vi "Event data  Queues Manager.vi"(0 "event":string, 1 "Mode":T1, 5 "Message":string, 7 "Time Stamp":timestamp, 9 "data":string, 11 "error in":errorcluster, 12 "Front?":bool) -> (6 "process":cluster{"event":string, "par":string}, 8 "data":cluster{"time":timestamp, "data":string}, 10 "timed out?":bool, 15 "error out":errorcluster)   [LabVIEW 2015, in "event data queues.lvlib"]
doc: "Use this template to build a VI to use as a subVI."
uses:
  event data queues.lvlib
  Enum data queue_Ctrls.ctl
panel:
  in  "queues":T2
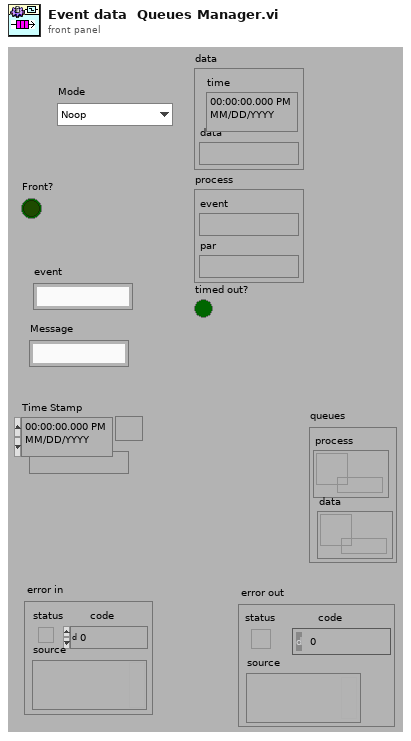
[diagram p1: front panel]
types:
  T1 = typedef "event data queues.lvlib/Enum data queue_Ctrls.ctl" = enum16{"Noop", "Send Pro1", "Send data", "Get Pro1", "Get data", "Flush Pro1", "Flush data", "Destroy Pro1", "Destroy data"}
  T2 = cluster{"process":refnum<queue>, "data":refnum<queue>}
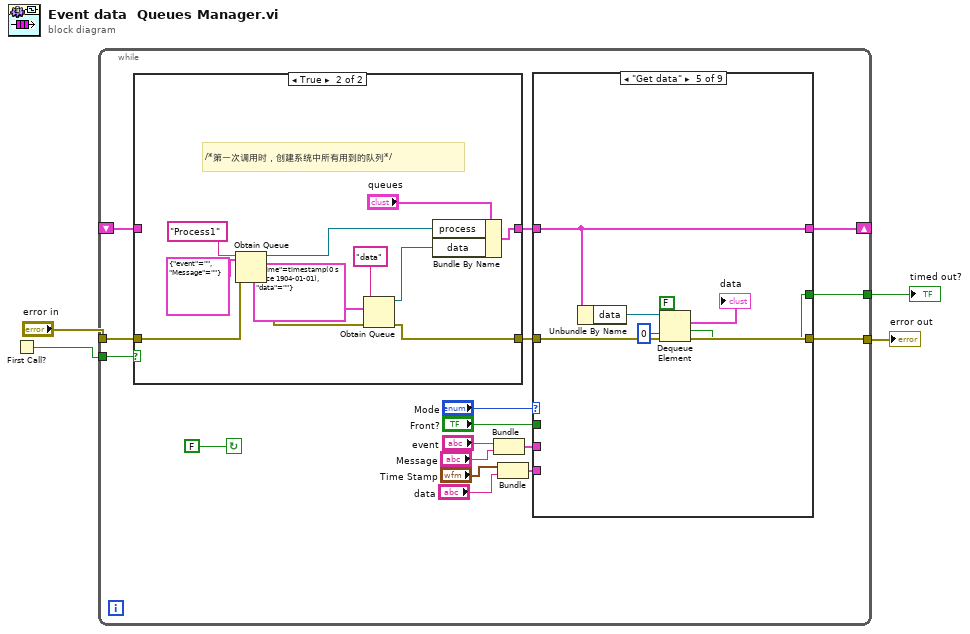
[diagram p0: block diagram]
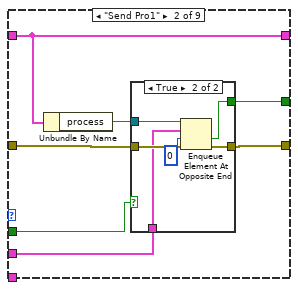
[diagram p3: hidden frame]
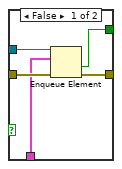
[diagram p4: hidden frame]
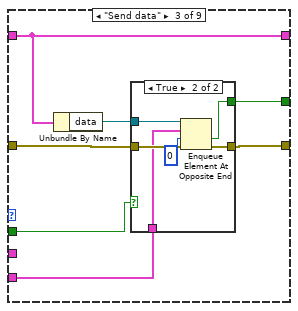
[diagram p5: hidden frame]
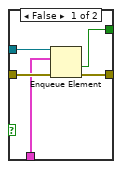
[diagram p6: hidden frame]
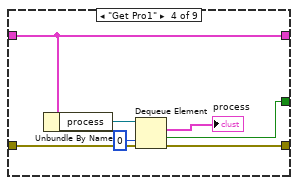
[diagram p7: hidden frame]
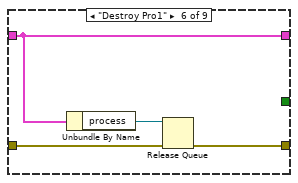
[diagram p8: hidden frame]
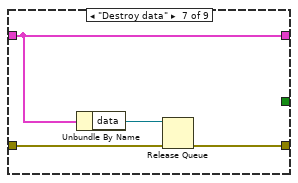
[diagram p9: hidden frame]
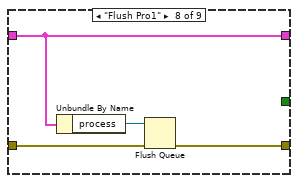
[diagram p10: hidden frame]
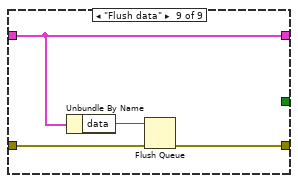
[diagram p11: hidden frame]
diagram:
  n1 = First Call?() -> (First Call?: T/F=w4:bool)
  n2 = while {
    tunnel: w4 -> [w20]
    tunnel: [w16] -> w2
    shift-right: [w15] -> _
    shift-left: _ -> [w14]
    tunnel: "error in" -> [w13]
    tunnel: [w5] -> w1
    stop <- FALSE continue-if-true
    n3 = case shown="True" w20 {
      tunnel: [w91 w100] -> w18
      tunnel: [w90 w97] -> w17
      tunnel: w14 -> [w91 _]
      tunnel: w13 -> [w90 w98]
      frame False {
      }
      frame True {
        # "/*第一次调用时，创建系统中所有用到的队列*/"
        n4 = Obtain Queue(name (unnamed)="Process1", element data type=cluster{"event":string, "Message":string} {"event"="", "Message"=""} ("Cluster"), error in (no error)=w98) -> (queue out=w93:refnum<queue>, error out=w94:errorcluster)  [unwired: 2 in, 1 out]
        n5 = Obtain Queue(name (unnamed)="data", element data type=cluster{"time":timestamp, "data":string} {"time"=timestamp(0 s since 1904-01-01), "data"=""} ("Cluster"), error in (no error)=w94) -> (queue out=w92:refnum<queue>, error out=w97:errorcluster)  [unwired: 2 in, 1 out]
        n6 = Bundle By Name(cluster="queues", "process"=w93, "data"=w92) -> (w100:T2)
      }
    }
    n7 = Bundle("event"="event", "Message"="Message") -> (w11:cluster{"event":string, "Message":string})  [unwired: 1 out]
    n8 = Bundle("Time Stamp"="Time Stamp", "data"="data") -> (w9:cluster{"Time Stamp":timestamp, "data":string})  [unwired: 1 out]
    n9 = case shown="\"Get data\"" "Mode" {
      tunnel: w18 -> [w23 w28 w46 w63 w70 w74 w78 w84 w88]
      tunnel: w17 -> [w22 w30 w48 w65 w72 w77 w81 w83 w87]
      tunnel: [w22 w29 w47 w64 w71 w76 w80 w82 w86] -> w16
      tunnel: [w23 w28 w46 w63 w70 w74 w78 w84 w88] -> w15
      tunnel: "Front?" -> [_ w27 w45 _ _ _ _ _ _]
      tunnel: w11 -> [_ w25 _ _ _ _ _ _ _]
      tunnel: w9 -> [_ _ w43 _ _ _ _ _ _]
      tunnel: [_ w24 w42 w60 w67 _ _ _ _] -> w5
      frame "Noop", Default {
      }
      frame "Send Pro1" {
        n10 = Unbundle By Name(w28) -> ("process"=w26:refnum<queue>)
        n11 = case shown="True" w27 {
          tunnel: w30 -> [w35 w41]
          tunnel: [w34 w40] -> w29
          tunnel: w26 -> [w33 w38]
          tunnel: w25 -> [w32 w37]
          tunnel: [w31 w36] -> w24
          frame False {
            n12 = Enqueue Element(queue=w33, element=w32, error in (no error)=w35) -> (timed out?=w31:bool, error out=w34:errorcluster)  [unwired: 2 out]
          }
          frame True {
            n13 = Enqueue Element At Opposite End(queue=w38, element=w37, timeout in ms (-1)=0, error in (no error)=w41) -> (timed out?=w36:bool, error out=w40:errorcluster)  [unwired: 1 out]
          }
        }
      }
      frame "Send data" {
        n14 = Unbundle By Name(w46) -> ("data"=w44:refnum<queue>)
        n15 = case shown="True" w45 {
          tunnel: w48 -> [w53 w59]
          tunnel: [w52 w58] -> w47
          tunnel: w44 -> [w51 w56]
          tunnel: w43 -> [w50 w55]
          tunnel: [w49 w54] -> w42
          frame False {
            n16 = Enqueue Element(queue=w51, element=w50, error in (no error)=w53) -> (timed out?=w49:bool, error out=w52:errorcluster)  [unwired: 1 in, 1 out]
          }
          frame True {
            n17 = Enqueue Element At Opposite End(queue=w56, element=w55, timeout in ms (-1)=0, error in (no error)=w59) -> (timed out?=w54:bool, error out=w58:errorcluster)  [unwired: 1 out]
          }
        }
      }
      frame "Get Pro1" {
        n18 = Unbundle By Name(w63) -> ("process"=w66:refnum<queue>)
        n19 = Dequeue Element(queue=w66, timeout in ms (-1)=0, error in (no error)=w65) -> (element=→"process":cluster{"event":string, "par":string}, timed out?=w60:bool, error out=w64:errorcluster)  [unwired: 1 out]
      }
      frame "Get data" {
        (unwired) FALSE ("timed out?")
        n20 = Unbundle By Name(w70) -> ("data"=w73:refnum<queue>)
        n21 = Dequeue Element(queue=w73, timeout in ms (-1)=0, error in (no error)=w72) -> (element=→"data":cluster{"time":timestamp, "data":string}, timed out?=w67:bool, error out=w71:errorcluster)  [unwired: 1 out]
      }
      frame "Destroy Pro1" {
        n22 = Unbundle By Name(w74) -> ("process"=w75:refnum<queue>)
        n23 = Release Queue(queue=w75, error in (no error)=w77) -> (error out=w76:errorcluster)  [unwired: 3 out]
      }
      frame "Destroy data" {
        n24 = Unbundle By Name(w78) -> ("data"=w79:refnum<queue>)
        n25 = Release Queue(queue=w79, error in (no error)=w81) -> (error out=w80:errorcluster)  [unwired: 3 out]
      }
      frame "Flush Pro1" {
        n26 = Unbundle By Name(w84) -> ("process"=w85:refnum<queue>)
        n27 = Flush Queue(queue=w85, error in (no error)=w83) -> (error out=w82:errorcluster)  [unwired: 2 out]
      }
      frame "Flush data" {
        n28 = Unbundle By Name(w88) -> ("data"=w89:refnum<queue>)
        n29 = Flush Queue(queue=w89, error in (no error)=w87) -> (error out=w86:errorcluster)  [unwired: 2 out]
      }
    }
  }
  "error out" <- w2
  "timed out?" <- w1
